vi "ExImageFileToSpreadsheet.vi"() -> ()   [LabVIEW 2010]
uses:
  <vilib>/Utility/file.llb/Write To Spreadsheet File (DBL).vi
panel:
  in  "2d Array Spreadsheet File Name (put in .xls on filename)":path
  in  "1d Array Spreadsheet File Name (put in .xls on filename)":path
  out "Test 2d Array":sgl[][](array[numeric]) format="%.2f"
  out "Test 1d array":sgl[](array[numeric]) format="%.2f"
  out "Pixel Value u16":u16
  out "Pixel Value i32":i32
  out "Pixel Value f32":sgl format="%.2f"
  out "error out":errorcluster
  in  "error in (no error)":errorcluster
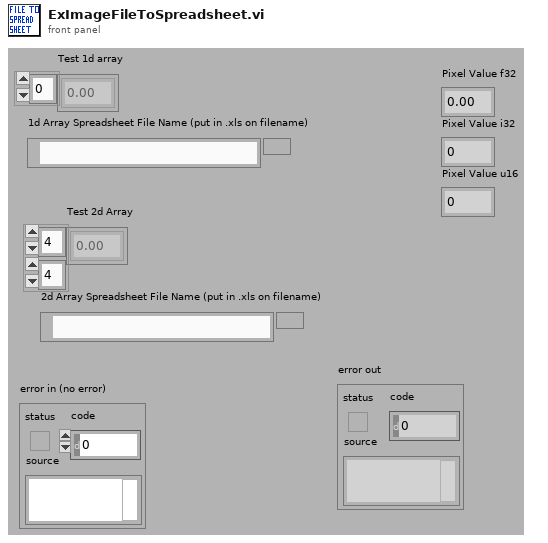
[diagram p1: front panel]
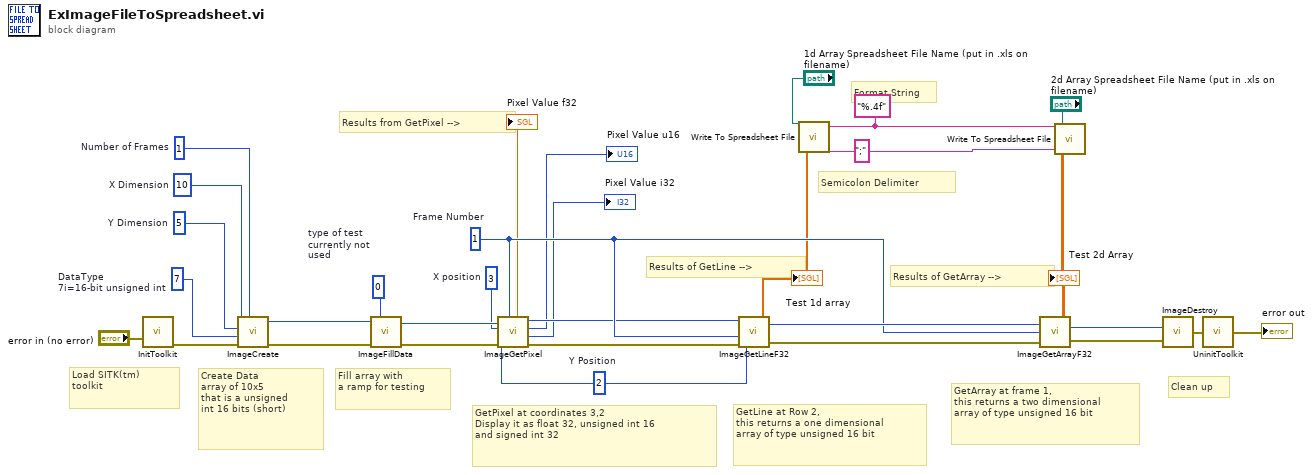
[diagram p0: block diagram]
diagram:
  w1 = ";"
  w2 = "%.4f"
  w12 = 1  # Frame Number
  w15 = 2  # Y Position
  w16 = 3  # X position
  w18 = 0  # type of test currently not used
  w20 = 1  # Number of Frames
  w21 = 10  # X Dimension
  w22 = 5  # Y Dimension
  w23 = 7  # DataType  7i=16-bit unsigned int
  # "Format String"
  # "Semicolon Delimiter"
  # "Clean up"
  # "Results of GetArray -->"
  # "GetArray at frame 1,\nthis returns a two dimensional\narray of type unsigned 16 bit"
  # "GetLine at Row 2,\nthis returns a one dimensional\narray of type unsigned 16 bit"
  # "Results of GetLine -->"
  # "GetPixel at coordinates 3,2\nDisplay it as float 32, unsigned int 16\nand signed int 32"
  # "Results from GetPixel -->"
  # "Fill array with \na ramp for testing"
  # "Create Data\narray of 10x5\nthat is a unsigned \nint 16 bits (short)"
  # "Load SITK(tm) \ntoolkit"
  n1 = call <userlib>:"InitToolkit.vi"("error in"="error in (no error)") -> ("error out"=w31:errorcluster)
  n2 = call <userlib>:"ImageCreate.vi"("X dimension"=w21, "Y dimension"=w22, "Data Type"=w23, "error in"=w31, "Number Of Frames"=w20) -> ("Image Handle"=w19:u32, "error out"=w27:errorcluster)
  n3 = call <userlib>:"ImageFillData.vi"("error in"=w27, "Type of Test"=w18, "Image Handle"=w19) -> ("error out"=w26:errorcluster, "Image Handle"=w17:u32)
  n4 = call <userlib>:"ImageGetPixel.vi"("Z position"=w12, "error in"=w26, "Y position"=w15, "X position"=w16, "Data Handle"=w17) -> ("error out"=w10:errorcluster, "Pixel Value i32"=→"Pixel Value i32":i32, "Pixel Value u16"=→"Pixel Value u16":u16, "Data Handle"=w11:u32, "Pixel Value f32"=→"Pixel Value f32":sgl)
  n5 = call <userlib>:"ImageGetLineF32.vi"("error in"=w10, "Z Position"=w12, "Y Position"=w15, "Data Handle"=w11) -> ("error out"=w25:errorcluster, "Array F32"=w6:sgl[], "Data Handle"=w14:u32)
  "Test 1d array" <- w6
  n6 = call-poly <vilib>:"Write To Spreadsheet File.vi"("delimiter (\\t)"=w1, "format (%.3f)"=w2, "1D data"=w6, "file path (dialog if empty)"="1d Array Spreadsheet File Name (put in .xls on filename)") -> ()  [unwired: 4 in, 1 out]
  n7 = call <userlib>:"ImageGetArrayF32.vi"("error in"=w25, "Z position"=w12, "Image Handle"=w14) -> ("error out"=w24:errorcluster, "Array Float 32"=w5:sgl[][], "Image Handle"=w13:u32)
  "Test 2d Array" <- w5
  n8 = call-poly <vilib>:"Write To Spreadsheet File.vi"("delimiter (\\t)"=w1, "format (%.3f)"=w2, "2D data"=w5, "file path (dialog if empty)"="2d Array Spreadsheet File Name (put in .xls on filename)") -> ()  [unwired: 4 in, 1 out]
  n9 = call <userlib>:"ImageDestroy.vi"("error in"=w24, "Data handle"=w13) -> ("error out"=w30:errorcluster)
  n10 = call <userlib>:"UninitToolkit.vi"("error in"=w30) -> ("error out"=→"error out":errorcluster)
